vi "NicmosComputeTiming.vi"(3 "Mask In [8x128x128]":bool[][][](array[boolean]), 9 "error in":errorcluster) -> (6 "error out":errorcluster)   [LabVIEW 2009]
uses:
  NicmosGlobal.vi
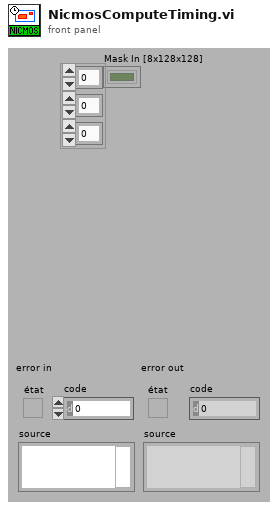
[diagram p1: front panel]
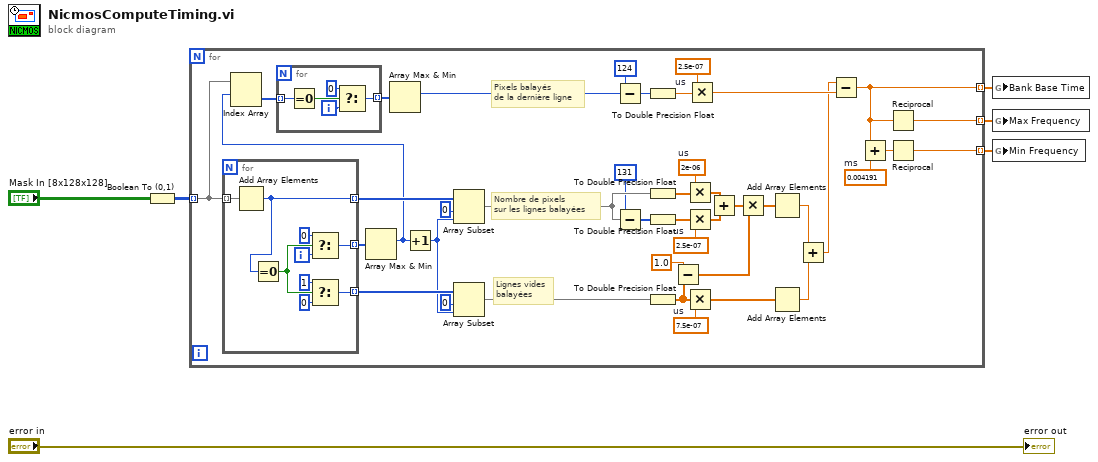
[diagram p0: block diagram]
diagram:
  n1 = Boolean To (0,1)(Boolean="Mask In [8x128x128]") -> (0, 1=w1:i16[][][])
  n2 = for {
    tunnel: w1 -> [w39] mode=indexing
    tunnel: [w11] -> w4 mode=indexing
    tunnel: [w8] -> w3 mode=indexing
    tunnel: [w7] -> w2 mode=indexing
    w10 = dbl[unit] 0.004191  # ms
    w22 = dbl[unit] 2.5e-07  # us
    w31 = dbl[unit] 2.5e-07  # us
    w35 = dbl[unit] 2e-06  # us
    w44 = dbl[unit] 7.5e-07  # us
    # "Pixels balayés\nde la dernière ligne"
    # "Nombre de pixels\nsur les lignes balayées"
    # "Lignes vides\nbalayées"
    n3 = for {
      tunnel: w39 -> [w61] mode=indexing
      tunnel: [w53] -> w47 mode=indexing
      tunnel: [w59] -> w46 mode=indexing
      tunnel: [w55] -> w42 mode=indexing
      i -> [w54]
      n4 = Add Array Elements(numeric array=w61) -> (sum=w53:i16)
      n5 = Equal To 0?(x=w53) -> (x = 0?=w56:bool)
      n6 = Select(t=0 ("cas vrai"), s=w56, f=w54) -> (s? t:f=w59:i32)
      n7 = Select(t=1 ("cas vrai"), s=w56, f=0 ("cas vrai")) -> (s? t:f=w55:i32)
    }
    n8 = Array Max & Min(array=w46) -> (max index (indices)=w36:i32)  [unwired: 3 out]
    n9 = Index Array(array=w39, index (row)=w36) -> (element=w38:i16[])  [unwired: 1 in]
    n10 = for {
      tunnel: w38 -> [w52] mode=indexing
      tunnel: [w48] -> w37 mode=indexing
      i -> [w49]
      n11 = Equal To 0?(x=w52) -> (x = 0?=w50:bool)
      n12 = Select(t=0 ("cas vrai"), s=w50, f=w49) -> (s? t:f=w48:i32)
    }
    n13 = Array Max & Min(array=w37) -> (max index (indices)=w19:i32)  [unwired: 3 out]
    n14 = Increment(x=w36) -> (x+1=w40:i32)
    n15 = Array Subset(array=w47, index=0 ("Indice du tableau"), length=w40) -> (w27:i16[])
    n16 = Array Subset(array=w42, index=0 ("Indice du tableau"), length=w40) -> (w41:i32[])
    n17 = Subtract(x=124, y=w19) -> (x-y=w18:i32)
    n18 = Subtract(x=131, y=w27) -> (x-y=w33:i32[])
    n19 = To Double Precision Float(number=w18) -> (double precision float=w21:dbl)
    n20 = To Double Precision Float(number=w27) -> (double precision float=w34:dbl[])
    n21 = To Double Precision Float(number=w33) -> (double precision float=w32:dbl[])
    n22 = To Double Precision Float(number=w41) -> (double precision float=w24:dbl[])
    n23 = Subtract(x=1.0, y=w24) -> (x-y=w23:dbl[])
    n24 = Multiply(x=w35, y=w34) -> (x*y=w30:dbl[unit][])
    n25 = Multiply(x=w32, y=w31) -> (x*y=w29:dbl[unit][])
    n26 = Multiply(x=w24, y=w44) -> (x*y=w16:dbl[unit][])
    n27 = Multiply(x=w22, y=w21) -> (x*y=w14:dbl[unit])
    n28 = Add(x=w30, y=w29) -> (x+y=w28:dbl[unit][])
    n29 = Multiply(x=w28, y=w23) -> (x*y=w17:dbl[unit][])
    n30 = Add Array Elements(numeric array=w17) -> (sum=w15:dbl[unit])
    n31 = Add Array Elements(numeric array=w16) -> (sum=w12:dbl[unit])
    n32 = Add(x=w15, y=w12) -> (x+y=w13:dbl[unit])
    n33 = Subtract(x=w13, y=w14) -> (x-y=w11:dbl[unit])
    n34 = Add(x=w11, y=w10) -> (x+y=w9:dbl[unit])
    n35 = Reciprocal(x=w11) -> (1/x=w8:dbl[unit])
    n36 = Reciprocal(x=w9) -> (1/x=w7:dbl[unit])
  }
  n37 = global write "NicmosGlobal.vi" "Bank Base Time"(w4) -> ()
  n38 = global write "NicmosGlobal.vi" "Max Frequency"(w3) -> ()
  n39 = global write "NicmosGlobal.vi" "Min Frequency"(w2) -> ()
  "error out" <- "error in"
